vi "Measure then Step Source.vi"(5 "Source Value (0.000)":dbl, 7 "Function (Current)":T1(ring), 8 "error in (no error)":errorcluster, 9 "Channel (Channel A)":T2, 10 "Node In":string, 11 "VISA resource name":refnum<visa-resource-name>) -> (0 "error out":errorcluster, 1 "Output":string, 2 "Node Out":string, 3 "VISA resource name out":refnum<visa-resource-name>, 4 "Command String":string)   [LabVIEW 2018, in "Keithley 2600 Series.lvlib"]
doc: "This VI performs one or two measurements and then steps the source.\n\n<b>Remarks:</b> Both source and measure auto range must be disabled before using this function.\n\n<b>Functions and Attributes Used</b>\nsmuX.measureYandstep(sourcevalue)\nsmuX.measureivandstep(sourcevalue)"
uses:
  Keithley 2600 Series.lvlib
  Private/GlobalVariables.vi
  Channel.ctl
panel:
  # "(c) 2008 Keithley Instruments, Inc.  ALL RIGHTS RESERVED."
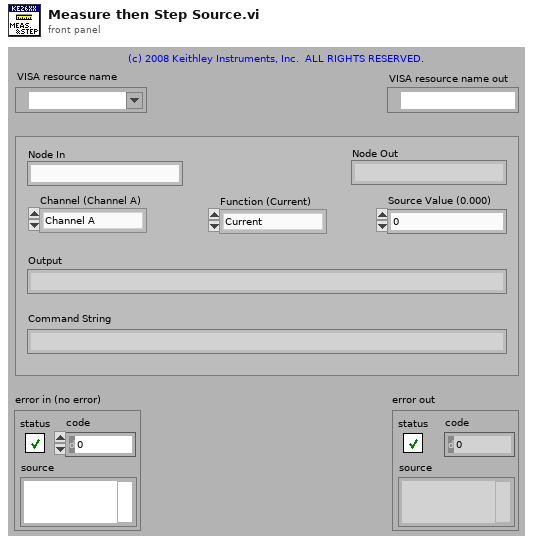
[diagram p1: front panel]
types:
  T1 = enum32{"Current", "Voltage", "IV", "Resistance", "Power"}
  T2 = typedef "Keithley 2600 Series.lvlib/Channel.ctl" = enum32{"Channel A", "Channel B"}
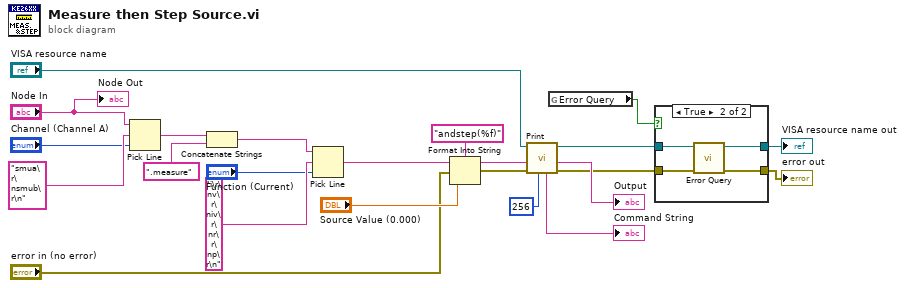
[diagram p0: block diagram]
diagram:
  n1 = Pick Line(string ("")="Node In", multi-line string="smua\r\nsmub\r\n" ("options"), line index="Channel (Channel A)") -> (output string=w22:string)
  n2 = Concatenate Strings(w22, ".measure" ("command")) -> (w20:string)
  n3 = Pick Line(string ("")=w20, multi-line string="i\r\nv\r\niv\r\nr\r\np\r\n" ("options"), line index="Function (Current)") -> (output string=w14:string)
  n4 = Format Into String(format string="andstep(%f)", initial string=w14, error in="error in (no error)", "Source Value (0.000)") -> (resulting string=w11:string, error out=w10:errorcluster)
  n5 = call "Print.vi"("Byte Count (1024)"=u32 256, "error in (no error)"=w10, "Input"=w11, "VISA resource name"="VISA resource name") -> ("error out"=w4:errorcluster, "Output"=→"Output":string, "VISA resource name out"=w5:refnum<visa-resource-name>, "Command String"=→"Command String":string)  [unwired: 1 in, 3 out]
  n6 = global read "GlobalVariables.vi" "Error Query"() -> (w6:bool)
  n7 = case shown="True" w6 {
    tunnel: w5 -> [w25 w29]
    tunnel: w4 -> [w24 w28]
    tunnel: [w25 w27] -> w3
    tunnel: [w24 w26] -> w2
    frame False {
    }
    frame True {
      n8 = call "Error Query.vi"("error in (no error)"=w28, "VISA resource name"=w29) -> ("error out"=w26:errorcluster, "VISA resource name out"=w27:refnum<visa-resource-name>)  [unwired: 8 out]
    }
  }
  "VISA resource name out" <- w3
  "error out" <- w2
  "Node Out" <- "Node In"
